vi "Find Frame Sink Terminal (Assuming only one sink).vi"(8 "error in (no error)":errorcluster, 9 "Frame Name":string, 11 "CaseStructure in":refnum<vi>) -> (0 "error IO":errorcluster, 1 "Found ?":bool, 2 "Terminal ref":refnum<vi>, 3 "CaseStructure out":refnum<vi>)   [LabVIEW 2019, in "gRPC Template Creation Utility.lvlib"]
uses:
  gRPC Template Creation Utility.lvlib
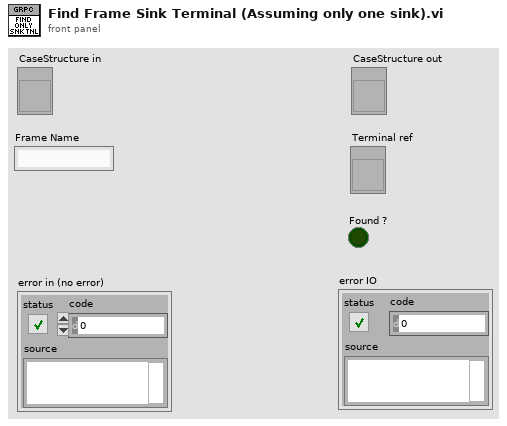
[diagram p1: front panel]
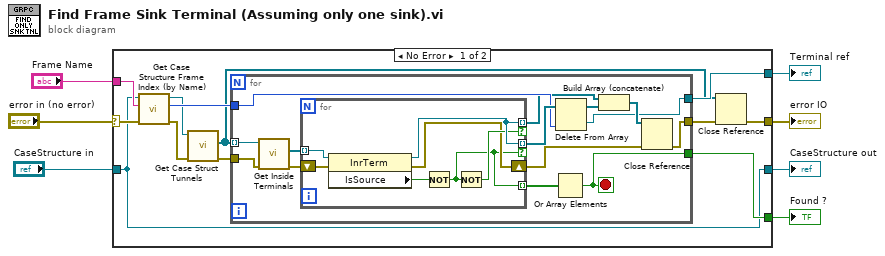
[diagram p0: block diagram]
diagram:
  n1 = case shown="No Error" "error in (no error)" {
    selector: "error in (no error)" -> [w14 w42]
    tunnel: "Frame Name" -> [w16 _]
    tunnel: "CaseStructure in" -> [w11 w41]
    tunnel: [w13 _] -> w3
    tunnel: [w12 _] -> w2
    tunnel: [w11 w41] -> w4
    tunnel: [w8 w42] -> w1
    frame No Error {
      n2 = call "Get Case Structure Frame Index (by Name).vi"("error in (no error)"=w14, "element"=w16, "CaseStructure in"=w11) -> ("error out"=w18:errorcluster, "Frame Index"=w19:i32, "CaseStructure out"=w17:refnum<vi>)  [unwired: 5 in, 1 out]
      n3 = call "Get Case Struct Tunnels.vi"("Error In"=w18, "Case Structure in"=w17) -> ("Error Out"=w15:errorcluster, "Tunnels[]"=w9:refnum<vi>[])  [unwired: 7 in, 1 out]
      n4 = for {
        tunnel: w15 -> [w33]
        tunnel: w9 -> [w32] mode=indexing
        tunnel: w19 -> [w28]
        tunnel: [w24] -> w13
        tunnel: [w22] -> w12
        tunnel: [w20] -> w10
        stop <- w22 stop-if-true
        n5 = call "Get Inside Terminals.vi"("Error In"=w33, "Tunnel in"=w32) -> ("Error Out"=w31:errorcluster, "InsideTerms[]"=w30:refnum<vi>[])  [unwired: 7 in, 1 out]
        n6 = for {
          tunnel: w30 -> [w40] mode=indexing
          tunnel: [w37] -> w29 mode=indexing if=w34
          tunnel: [w37] -> w27 mode=indexing if=w36
          tunnel: [w34] -> w23 mode=indexing
          shift-right: [w35] -> w21
          shift-left: w31 -> [w38]
          n7 = property class="InrTerm"(reference=w40, error in=w38) -> (reference out=w37:refnum<vi>, error out=w35:errorcluster, "IsSource"=w39:bool)
          n8 = Not(x=w39) -> (.not. x?=w34:bool)
          n9 = Not(x=w34) -> (.not. x?=w36:bool)
        }
        n10 = Or Array Elements(Boolean array=w23) -> (logical OR=w22:bool)
        n11 = Delete From Array(array=w29, index=w28) -> (deleted portion=w24:refnum<vi>, array with subset deleted=w26:refnum<vi>[])  [unwired: 1 in]
        n12 = Build Array (concatenate)(w27, w26) -> (w25:refnum<vi>[])
        n13 = Close Reference(reference=w25, error in (no error)=w21) -> (error out=w20:errorcluster)
      }
      n14 = Close Reference(reference=w9, error in (no error)=w10) -> (error out=w8:errorcluster)
    }
    frame Error {
    }
  }
  "CaseStructure out" <- w4
  "Terminal ref" <- w3
  "Found ?" <- w2
  "error IO" <- w1
